vi "SPI Write Read.vi"   [LabVIEW 2014, in "LMH-LINX.lvlib"]
uses:
  <vilib>/MakerHub/LINX/LMH-LINX.lvlib
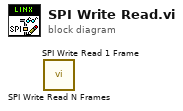
[diagram p0: block diagram]
diagram:
  n1 = call <vilib>:"SPI Write Read N Frames.vi"() -> ()  [unwired: 9 in, 3 out]
  n2 = call <vilib>:"SPI Write Read 1 Frame.vi"() -> ()  [unwired: 9 in, 3 out]
